vi "Focus BP.vi"(8 "error in":errorcluster, 9 "Scan Inc":dbl=0.01 format="%#_13g", 10 "Start Inc":dbl=-1.0 format="%#_13g", 11 "Gantry In":refnum<k24>) -> (0 "error out":errorcluster, 2 "max value":dbl, 3 "Gantry Out":refnum<k24>)   [LabVIEW 2021, in "Assembly Tray.lvclass"]
uses:
  Assembly Tray.lvclass
  C:/Program Files (x86)/Aerotech/A3200/LabVIEW/2010/Bin/Aerotech.A3200.dll
  Program Files (x86)/Aerotech/A3200/LabVIEW/2010/Bin/Aerotech.A3200.dll
  Controller/Motion/A3200/A3200.lvclass
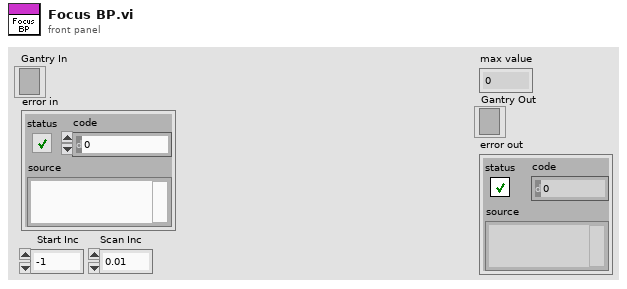
[diagram p1: front panel]
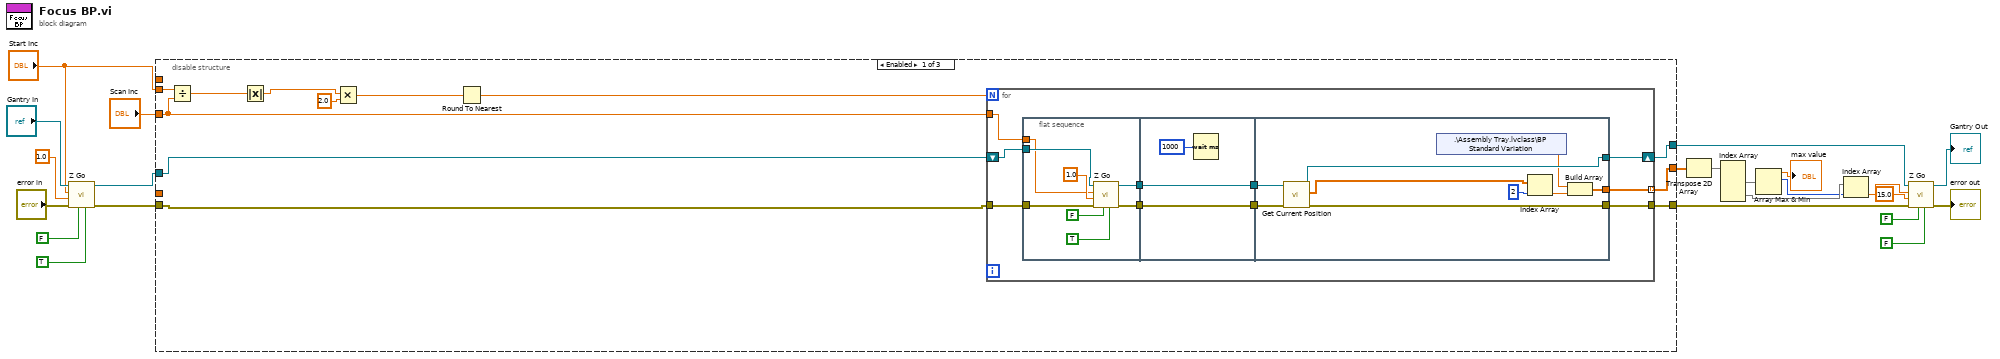
[diagram p0: block diagram]
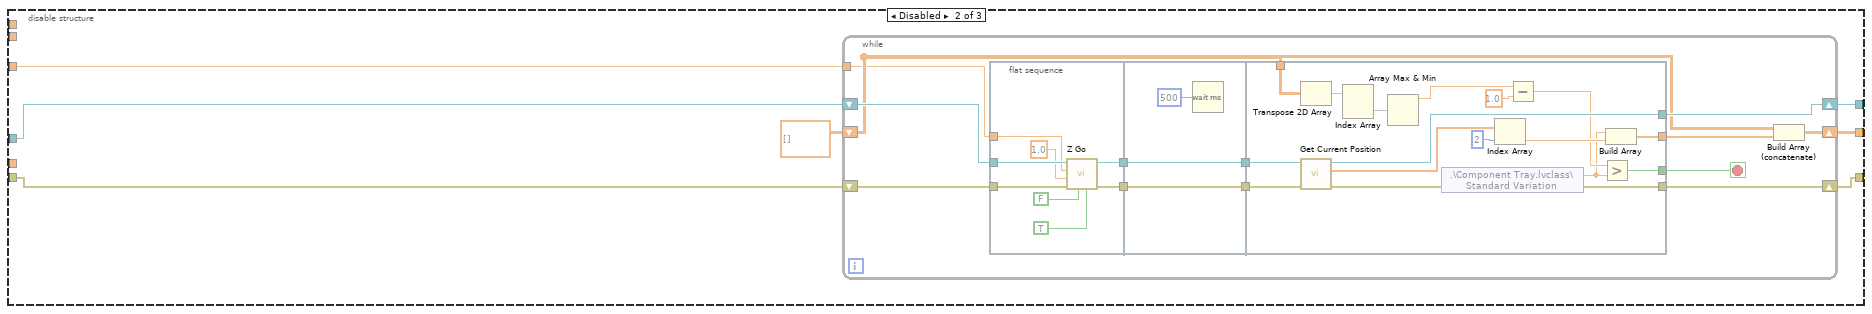
[diagram p2: hidden frame]
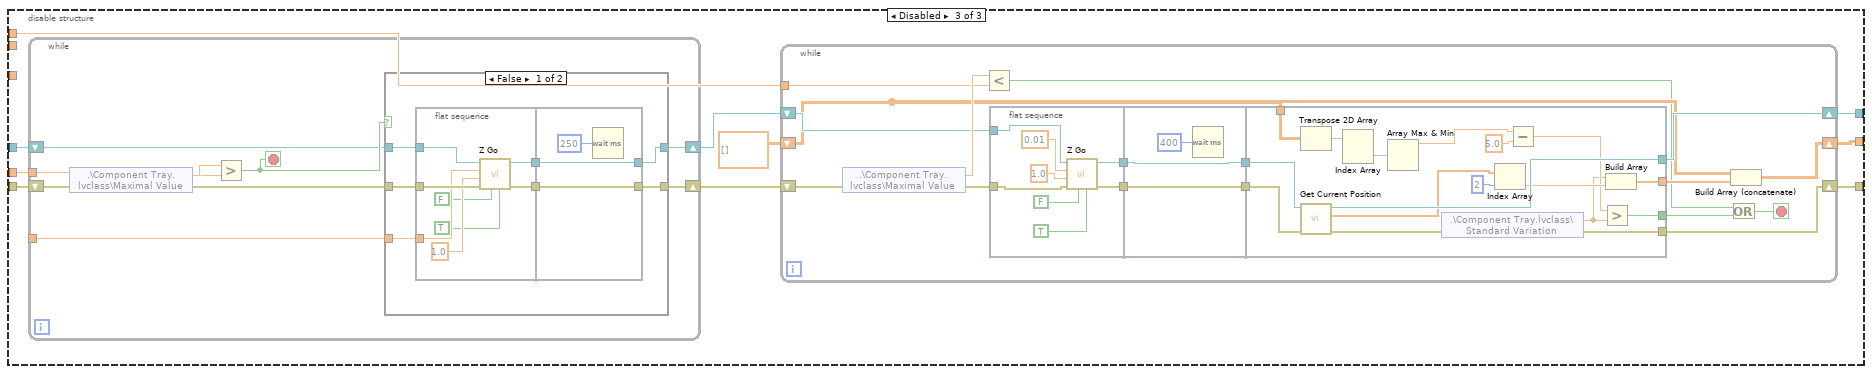
[diagram p3: hidden frame]
diagram:
  n1 = call "Z Go.vi"("Increment"=TRUE, "Return Immediately"=FALSE ("Increment"), "error in (no error)"="error in", "Speed In"=1.0 ("Speed"), "Position In"="Start Inc", "Gantry In"="Gantry In") -> ("error out"=w5:errorcluster, "Gantry Out"=w6:refnum<k24>)  [unwired: 2 in, 2 out]
  n2 = disable-structure shown="Enabled" {
    disable-tunnel: [w35 w68 w117] -> w20
    disable-tunnel: [w34 w69 w118] -> w17
    disable-tunnel: [w33 w70 w120] -> w16
    disable-tunnel: w6 -> [w32 w72 w123]
    disable-tunnel: w5 -> [w24 w71 w122]
    disable-tunnel: _ -> [_ _ w115]
    disable-tunnel: _ -> [_ _ w114]
    disable-tunnel: "Scan Inc" -> [w30 w66 _]
    disable-tunnel: "Start Inc" -> [w31 _ _]
    frame Enabled {
      n3 = Divide(x=w31, y=w30) -> (x/y=w28:dbl)
      n4 = Absolute Value(x=w28) -> (abs(x)=w27:dbl)
      n5 = Multiply(x=w27, y=2.0) -> (x*y=w26:dbl)
      n6 = Round To Nearest(number=w26) -> (nearest integer value=w25:dbl)
      n7 = for {
        N: w25 -> [_]
        tunnel: [w43] -> w35 mode=indexing
        tunnel: w24 -> [w42]
        tunnel: [w41] -> w33
        shift-right: [w44] -> w34
        shift-left: w32 -> [w45]
        tunnel: w30 -> [w36]
        n8 = flat-sequence {
          tunnel: w45 -> [w53]
          tunnel: [w52] -> w40
          tunnel: w42 -> [w51]
          tunnel: [w50] -> w38
          tunnel: w36 -> [w48]
          tunnel: w40 -> [w56]
          tunnel: [w56] -> w39
          tunnel: w38 -> [w55]
          tunnel: [w55] -> w37
          tunnel: w39 -> [w65]
          tunnel: [w64] -> w44
          tunnel: [w63] -> w43
          tunnel: w37 -> [w62]
          tunnel: [w61] -> w41
          frame #0 {
            n9 = call "Z Go.vi"("Increment"=TRUE, "Return Immediately"=FALSE ("Increment"), "error in (no error)"=w51, "Speed In"=1.0 ("Speed"), "Position In"=w48, "Gantry In"=w53) -> ("error out"=w50:errorcluster, "Gantry Out"=w52:refnum<k24>)  [unwired: 2 in, 2 out]
          }
          frame #1 {
            n10 = Wait (ms)(milliseconds to wait=u32 1000) -> ()  [unwired: 1 out]
          }
          frame #2 {
            n11 = call "Get Current Position.vi"("error in (no error)"=w62, "Gantry In"=w65) -> ("error out"=w61:errorcluster, "XYZTheta Out"=w60:dbl[], "Gantry Out"=w64:refnum<k24>)  [unwired: 7 in]
            n12 = shared-variable ".\\Assembly Tray.lvclass\\BP Standard Variation"() -> (w57:sgl)  [unwired: 1 in, 1 out]
            n13 = Index Array(array=w60, index=2) -> (element=w58:dbl)
            n14 = Build Array(w57, w58) -> (w63:dbl[])
          }
        }
      }
    }
    frame Disabled {
      n15 = while {
        shift-right: [w77] -> w68
        shift-left: dbl[][] [] -> [w76]
        shift-right: [w83] -> w69
        shift-left: w72 -> [w84]
        shift-right: [w85] -> w70
        shift-left: w71 -> [w74]
        tunnel: w66 -> [w73]
        stop <- w75 stop-if-true
        n16 = flat-sequence {
          tunnel: w84 -> [w93]
          tunnel: [w92] -> w82
          tunnel: w74 -> [w91]
          tunnel: [w90] -> w81
          tunnel: w73 -> [w86]
          tunnel: w82 -> [w96]
          tunnel: [w96] -> w80
          tunnel: w81 -> [w95]
          tunnel: [w95] -> w79
          tunnel: w80 -> [w113]
          tunnel: [w112] -> w83
          tunnel: [w111] -> w78
          tunnel: w79 -> [w107]
          tunnel: [w105] -> w85
          tunnel: w76 -> [w104]
          tunnel: [w97] -> w75
          frame #0 {
            n17 = call "Z Go.vi"("Increment"=TRUE, "Return Immediately"=FALSE ("Increment"), "error in (no error)"=w91, "Speed In"=1.0 ("Speed"), "Position In"=w86, "Gantry In"=w93) -> ("error out"=w90:errorcluster, "Gantry Out"=w92:refnum<k24>)  [unwired: 2 in, 2 out]
          }
          frame #1 {
            n18 = Wait (ms)(milliseconds to wait=u32 500) -> ()  [unwired: 1 out]
          }
          frame #2 {
            n19 = Transpose 2D Array(2D array=w104) -> (transposed array=w103:dbl[][])
            n20 = call "Get Current Position.vi"("error in (no error)"=w107, "Gantry In"=w113) -> ("error out"=w106:errorcluster, "XYZTheta Out"=w110:dbl[], "Gantry Out"=w112:refnum<k24>)  [unwired: 7 in]
            n21 = Index Array(array=w103) -> (element=w102:dbl[])  [unwired: 2 in]
            n22 = Array Max & Min(array=w102) -> (max value=w101:dbl)  [unwired: 3 out]
            n23 = shared-variable ".\\Component Tray.lvclass\\Standard Variation"(error in=w106) -> (w98:sgl, error out=w105:errorcluster)
            n24 = Index Array(array=w110, index=2) -> (element=w108:dbl)
            n25 = Subtract(x=w101, y=1.0) -> (x-y=w99:dbl)
            n26 = Greater?(x=w99, y=w98) -> (0:w97:bool)
            n27 = Build Array(w98, w108) -> (w111:dbl[])
          }
        }
        n28 = Build Array (concatenate)(w76, w78) -> (w77:dbl[][])
      }
    }
    frame Disabled {
      n29 = while {
        shift-right: [w174] -> w119
        shift-left: w123 -> [w175]
        shift-right: [w173] -> w121
        shift-left: w122 -> [w171]
        tunnel: _ -> [w172]
        tunnel: w115 -> [w169]
        stop <- w176 stop-if-true
        n30 = shared-variable ".\\Component Tray.lvclass\\Maximal Value"(error in=w171) -> (w177:sgl, error out=w170:errorcluster)
        n31 = Greater?(x=w177, y=w169) -> (0:w176:bool)
        n32 = case shown="False" w176 {
          tunnel: w175 -> [w182 w197]
          tunnel: [w179 w197] -> w174
          tunnel: [w178 w196] -> w173
          tunnel: w170 -> [w181 w196]
          tunnel: w172 -> [w180 _]
          frame False {
            n33 = flat-sequence {
              tunnel: w182 -> [w192]
              tunnel: [w191] -> w184
              tunnel: w181 -> [w190]
              tunnel: [w189] -> w183
              tunnel: w180 -> [w187]
              tunnel: w184 -> [w194]
              tunnel: w183 -> [w193]
              tunnel: [w194] -> w179
              tunnel: [w193] -> w178
              frame #0 {
                n34 = call "Z Go.vi"("Increment"=TRUE, "Return Immediately"=FALSE ("Increment"), "error in (no error)"=w190, "Speed In"=1.0 ("Speed"), "Position In"=w187, "Gantry In"=w192) -> ("error out"=w189:errorcluster, "Gantry Out"=w191:refnum<k24>)  [unwired: 2 in, 2 out]
              }
              frame #1 {
                n35 = Wait (ms)(milliseconds to wait=u32 250) -> ()  [unwired: 1 out]
              }
            }
          }
          frame True {
          }
        }
      }
      n36 = while {
        shift-right: [w129] -> w117
        shift-left: dbl[][] [] -> [w127]
        tunnel: w114 -> [w128]
        shift-right: [w137] -> w118
        shift-left: w119 -> [w138]
        shift-right: [w139] -> w120
        shift-left: w121 -> [w136]
        stop <- w125 stop-if-true
        n37 = shared-variable ".\\Component Tray.lvclass\\Maximal Value"(error in=w136) -> (w140:sgl, error out=w135:errorcluster)
        n38 = Less?(x=w140, y=w128) -> (x < y?=w126:bool)
        n39 = flat-sequence {
          tunnel: w138 -> [w148]
          tunnel: [w147] -> w134
          tunnel: w135 -> [w146]
          tunnel: [w145] -> w133
          tunnel: w134 -> [w151]
          tunnel: [w151] -> w132
          tunnel: w133 -> [w150]
          tunnel: [w150] -> w131
          tunnel: w132 -> [w168]
          tunnel: [w167] -> w137
          tunnel: [w166] -> w130
          tunnel: w131 -> [w162]
          tunnel: [w160] -> w139
          tunnel: w127 -> [w159]
          tunnel: [w152] -> w124
          frame #0 {
            n40 = call "Z Go.vi"("Increment"=TRUE, "Return Immediately"=FALSE ("Increment"), "error in (no error)"=w146, "Speed In"=1.0 ("Speed"), "Position In"=0.01, "Gantry In"=w148) -> ("error out"=w145:errorcluster, "Gantry Out"=w147:refnum<k24>)  [unwired: 2 in, 2 out]
          }
          frame #1 {
            n41 = Wait (ms)(milliseconds to wait=u32 400) -> ()  [unwired: 1 out]
          }
          frame #2 {
            n42 = Transpose 2D Array(2D array=w159) -> (transposed array=w158:dbl[][])
            n43 = call "Get Current Position.vi"("error in (no error)"=w162, "Gantry In"=w168) -> ("error out"=w161:errorcluster, "XYZTheta Out"=w165:dbl[], "Gantry Out"=w167:refnum<k24>)  [unwired: 7 in]
            n44 = Index Array(array=w158) -> (element=w157:dbl[])  [unwired: 2 in]
            n45 = Array Max & Min(array=w157) -> (max value=w156:dbl)  [unwired: 3 out]
            n46 = shared-variable ".\\Component Tray.lvclass\\Standard Variation"(error in=w161) -> (w153:sgl, error out=w160:errorcluster)
            n47 = Index Array(array=w165, index=2) -> (element=w163:dbl)
            n48 = Subtract(x=w156, y=5.0) -> (x-y=w154:dbl)
            n49 = Greater?(x=w154, y=w153) -> (0:w152:bool)
            n50 = Build Array(w153, w163) -> (w166:dbl[])
          }
        }
        n51 = Or(x=w126, y=w124) -> (x .or. y?=w125:bool)
        n52 = Build Array (concatenate)(w127, w130) -> (w129:dbl[][])
      }
    }
  }
  n53 = Transpose 2D Array(2D array=w20) -> (transposed array=w10:dbl[][])
  n54 = Index Array(array=w10) -> (element #1=w7:dbl[], element #2=w9:dbl[])  [unwired: 4 in]
  n55 = Array Max & Min(array=w7) -> (max value=→"max value":dbl, max index (indices)=w8:i32)  [unwired: 2 out]
  n56 = Index Array(array=w9, index=w8) -> (element=w19:dbl)
  n57 = call "Z Go.vi"("Increment"=FALSE, "Return Immediately"=FALSE ("Increment"), "error in (no error)"=w16, "Speed In"=15.0 ("Speed"), "Position In"=w19, "Gantry In"=w17) -> ("error out"=→"error out":errorcluster, "Gantry Out"=→"Gantry Out":refnum<k24>)  [unwired: 2 in, 2 out]
